vi "PXI-DAQ loop stop test.vi"(7 "Cycle":i32, 11 "error in (no error)":errorcluster, 12 "DAQ Write State":T1) -> (8 "Stop?":bool, 14 "DAQ Write State out":T1, 15 "error out":errorcluster)   [LabVIEW 2020]
uses:
  Type Defs/DAQ Write State enum.ctl
  PXI Globals.vi
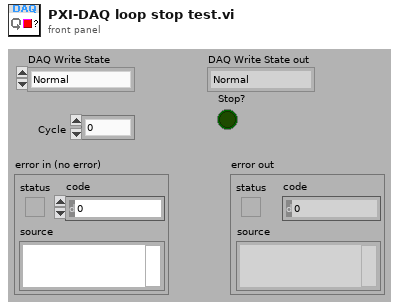
[diagram p1: front panel]
types:
  T1 = typedef "DAQ Write State enum.ctl" = enum16{"Normal", "Ramp down", "Zero buffers", "Done"}
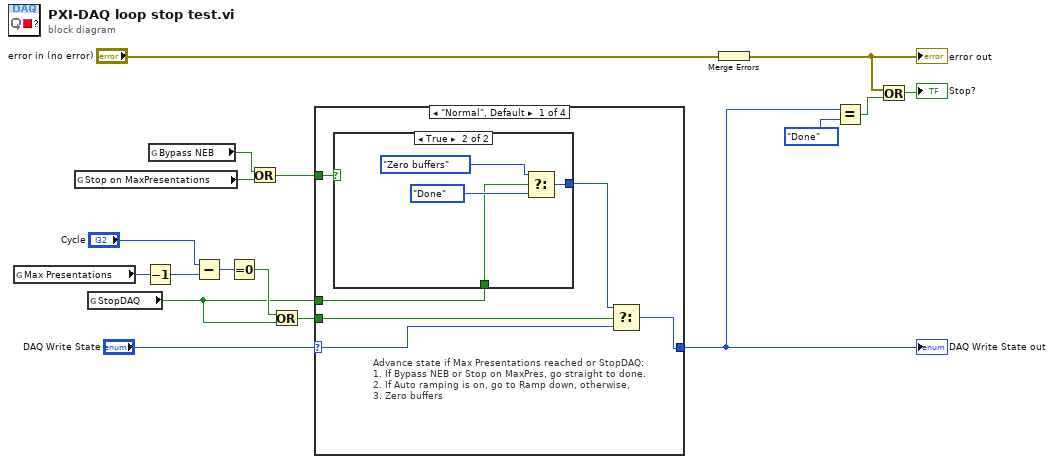
[diagram p0: block diagram]
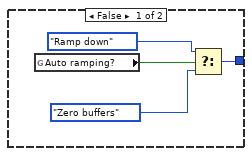
[diagram p2: hidden frame]
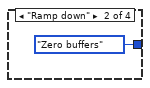
[diagram p3: hidden frame]
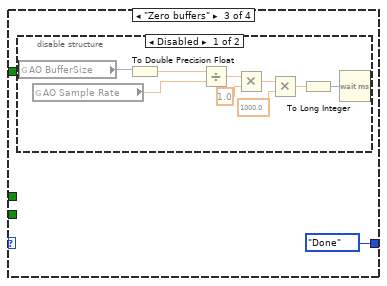
[diagram p4: hidden frame]
diagram:
  n1 = global read "PXI Globals.vi" "Max Presentations"() -> (w17:i32)
  n2 = global read "PXI Globals.vi" "Stop on MaxPresentations"() -> (w14:bool)
  n3 = global read "PXI Globals.vi" "StopDAQ"() -> (w1:bool)
  n4 = Decrement(x=w17) -> (x-1=w16:i32)
  n5 = global read "PXI Globals.vi" "Bypass NEB"() -> (w12:bool)
  n6 = Subtract(x="Cycle", y=w16) -> (x-y=w11:i32)
  n7 = Equal To 0?(x=w11) -> (x = 0?=w9:bool)
  n8 = Or(x=w12, y=w14) -> (x .or. y?=w5:bool)
  n9 = Or(x=w9, y=w1) -> (x .or. y?=w8:bool)
  n10 = case shown="\"Normal\", Default" "DAQ Write State" {
    selector: "DAQ Write State" -> [w23 _ _ w43]
    tunnel: w8 -> [w20 _ _ _]
    tunnel: [w19 DAQ_Write_State_enum."Zero buffers" ("DAQ Write State") DAQ_Write_State_enum."Done" ("DAQ Write State") w43] -> w4
    tunnel: w5 -> [w21 _ _ _]
    tunnel: w1 -> [w18 _ _ _]
    frame "Normal", Default {
      # "Advance state if Max Presentations reached or StopDAQ:\n1. If Bypass NEB or Stop on MaxPres, go straight to done.\n2. If Auto ramping is on, go to Ramp down, otherwise,\n3. Zero buffers"
      n11 = case shown="True" w21 {
        tunnel: [w25 w28] -> w22
        tunnel: w18 -> [_ w29]
        frame False {
          n12 = global read "PXI Globals.vi" "Auto ramping?"() -> (w24:bool)
          n13 = Select(t=DAQ_Write_State_enum."Ramp down", s=w24, f=DAQ_Write_State_enum."Zero buffers") -> (s? t:f=w25:T1)
        }
        frame True {
          n14 = Select(t=DAQ_Write_State_enum."Zero buffers", s=w29, f=DAQ_Write_State_enum."Done") -> (s? t:f=w28:T1)
        }
      }
      n15 = Select(t=w22, s=w20, f=w23) -> (s? t:f=w19:T1)
    }
    frame "Ramp down" {
    }
    frame "Zero buffers" {
      n16 = disable-structure shown="Disabled" {
        frame Disabled {
          n17 = global read "PXI Globals.vi" "AO BufferSize"() -> (w35:i32)
          n18 = global read "PXI Globals.vi" "AO Sample Rate"() -> (w42:dbl)
          n19 = To Double Precision Float(number=w35) -> (double precision float=w41:dbl)
          n20 = Divide(x=w41, y=w42) -> (x/y=w40:dbl)
          n21 = Multiply(x=w40, y=1.0) -> (x*y=w38:dbl)
          n22 = Multiply(x=w38, y=1000.0) -> (x*y=w36:dbl)
          n23 = To Long Integer(number=w36) -> (32bit integer=w34:i32)
          n24 = Wait (ms)(milliseconds to wait=w34) -> ()  [unwired: 1 out]
        }
        frame Enabled {
        }
      }
    }
    frame "Done" {
    }
  }
  "DAQ Write State out" <- w4
  n25 = Merge Errors("error in (no error)") -> (w2:errorcluster)
  "error out" <- w2
  n26 = Equal?(x=w4, y=DAQ_Write_State_enum."Done" ("x")) -> (x = y?=w7:bool)
  n27 = Or(x=w2, y=w7) -> (x .or. y?=→"Stop?":bool)
